vi "ReadCount.vi"(11 "TypedCircularBuffer in":refnum<class "LogCircularBuffer.lvclass">) -> (2 "Count":u32, 3 "TypedCircularBuffer out":refnum<class "LogCircularBuffer.lvclass">)   [LabVIEW 2024, in "LogCircularBuffer.lvclass"]
uses:
  LogCircularBuffer.lvclass
  LogCircularBuffer.lvclass/LogCircularBuffer.ctl
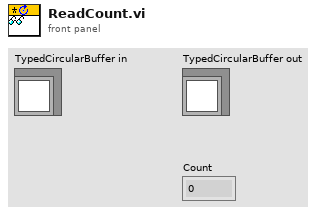
[diagram p1: front panel]
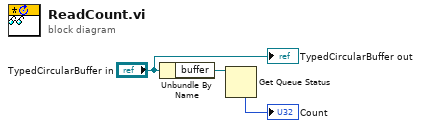
[diagram p0: block diagram]
diagram:
  n1 = Unbundle By Name("TypedCircularBuffer in") -> ("buffer"=w2:refnum<queue>)
  n2 = Get Queue Status(queue=w2) -> (# elements in queue=→"Count":i32)  [unwired: 2 in, 7 out]
  "TypedCircularBuffer out" <- "TypedCircularBuffer in"
